vi "IQ_Trim_CP.vi"(11 "IQ_With_CP":cdb[](array[numeric])=array[30720 elements]) -> (3 "IQ_NO_CP":cdb[](array[numeric]))   [LabVIEW 2015]
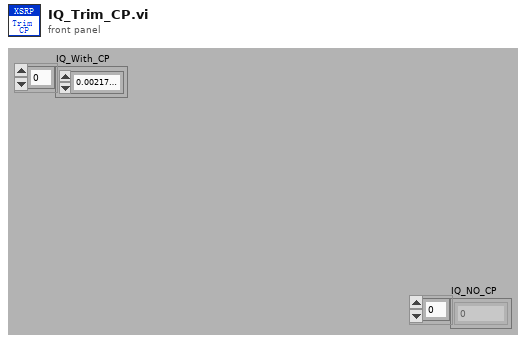
[diagram p1: front panel]
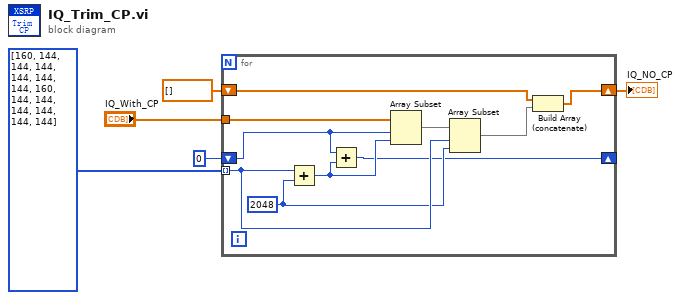
[diagram p0: block diagram]
diagram:
  n1 = for {
    tunnel: "IQ_With_CP" -> [w15]
    shift-right: [w14] -> w2
    shift-left: dbl[] [] -> [w13]
    tunnel: i32[] [160, 144, 144, 144, 144, 144, 144, 160, 144, 144, 144, 144, 144, 144] -> [w11] mode=indexing
    shift-right: [w6] -> _
    shift-left: 0 -> [w8]
    w10 = 2048 ("x")
    n2 = Add(x=w11, y=w10) -> (x+y=w7:i32)
    n3 = Add(x=w8, y=w7) -> (x+y=w6:i32)
    n4 = Array Subset(array=w15, index=w8, length=w7) -> (w12:cdb[])
    n5 = Array Subset(array=w12, index=w11, length=w10) -> (w9:cdb[])
    n6 = Build Array (concatenate)(w13, w9) -> (w14:cdb[])
  }
  "IQ_NO_CP" <- w2
